vi "SHO solver.vi"() -> ()   [LabVIEW 2015]
uses:
  <vilib>/Simulation/Utility/Implementation/Shared/SIM Diagram Parameters.ctl
  <vilib>/Simulation/Implementation/Shared/SIM Continuous Solvers.ctl
  <vilib>/gmath/ode.llb/ODE Solver main.vi
  <vilib>/gmath/NI_Gmath.lvlib
panel:
  out "radius vs t plot":cluster{"outputs":dbl[], "outputs":dbl[]}(graph)
  out "sqrt(x)":dbl[](array[numeric])
  out "v vs x plot":cluster{"outputs":dbl[], "outputs":dbl[]}(graph)
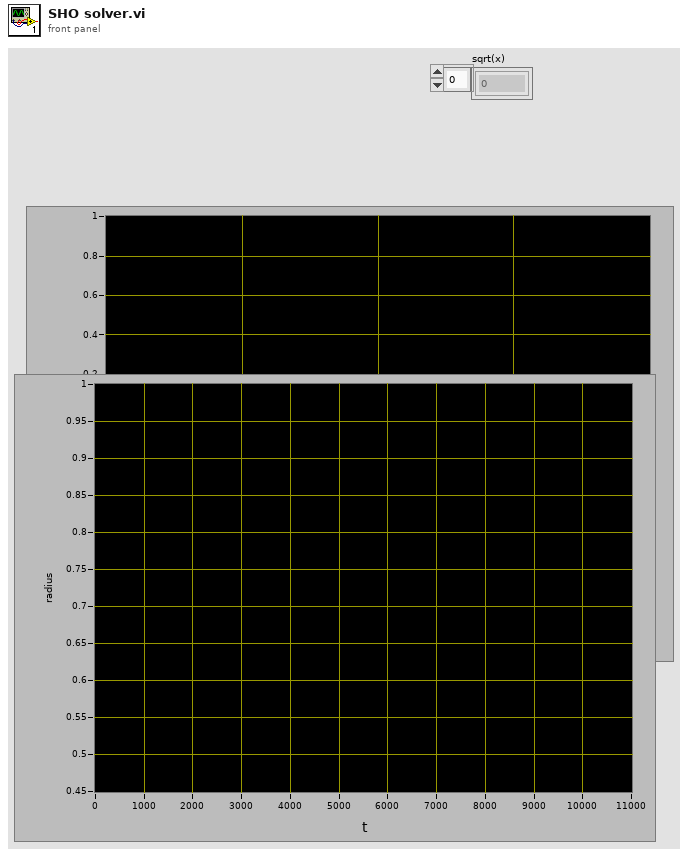
[diagram p1: front panel]
types:
  T1 = typedef "SIM Continuous Solvers.ctl" = enum16{"Runge-Kutta 1 (Euler)", "Runge-Kutta 2", "Runge-Kutta 3", "Runge-Kutta 4", "Runge-Kutta 23 (variable)", "Runge-Kutta 45 (variable)", "BDF (variable)", "Adams-Moulton (variable)", "Rosenbrock (variable)", "Discrete States Only"}
  T2 = typedef "SIM Diagram Parameters.ctl" = cluster{"Initial Time":dbl, "Final Time":dbl, "Time Step":dbl, "Absolute Tolerance":dbl, "Relative Tolerance":dbl, "Continuous Solver":T1, "Discrete Time Step":dbl, "Minimum Time Step":dbl, "Maximum Time Step":dbl, "Initial Time Step":dbl}
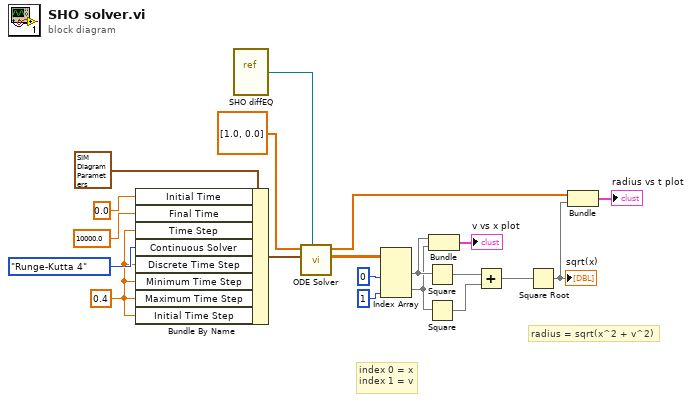
[diagram p0: block diagram]
diagram:
  w9 = 0.4 ("Time Step")
  # "radius = sqrt(x^2 + v^2)"
  # "index 0 = x\nindex 1 = v"
  n1 = Bundle By Name(cluster=T2 {"Initial Time"=0.0, "Final Time"=10.0, "Time Step"=0.1, "Absolute Tolerance"=0.001, "Relative Tolerance"=0.001, "Continuous Solver"=enum."Runge-Kutta 45 (variable)", "Discrete Time Step"=1.0, "Minimum Time Step"=1e-08, "Maximum Time Step"=1.0, "Initial Time Step"=0.01} ("simulation parameters"), "Initial Time"=0.0, "Final Time"=10000.0, "Time Step"=w9, "Continuous Solver"=SIM_Continuous_Solvers."Runge-Kutta 4", "Discrete Time Step"=w9, "Minimum Time Step"=w9, "Maximum Time Step"=w9, "Initial Time Step"=w9) -> (w15:T2)
  n2 = vi-ref "SHO diffEQ.vi"() -> ("vi reference"=w14:refnum<vi>)
  n3 = call-poly <vilib>:"ODE Solver.vi"("ODE F(X,t)"=w14, "simulation parameters"=w15, "x0"=dbl[] [1.0, 0.0]) -> ("outputs"=w13:dbl[][], "times"=w3:dbl[])  [unwired: 6 in, 1 out]
  n4 = Index Array(array=w13, index (col) #1=0 ("disabled index (col)"), index (col) #2=1 ("index (col)")) -> (element #1=w8:dbl[], element #2=w7:dbl[])  [unwired: 2 in]
  n5 = Square(x=w8) -> (x^2=w6:dbl[])
  n6 = Square(x=w7) -> (x^2=w5:dbl[])
  n7 = Bundle("outputs"=w8, "outputs"=w7) -> (→"v vs x plot":cluster{"outputs":dbl[], "outputs":dbl[]})  [unwired: 1 in]
  n8 = Add(x=w6, y=w5) -> (x+y=w4:dbl[])
  n9 = Square Root(x=w4) -> (sqrt(x)=w2:dbl[])
  "sqrt(x)" <- w2
  n10 = Bundle("times"=w3, w2) -> (→"radius vs t plot":cluster{"times":dbl[], dbl[]})  [unwired: 1 in]
